vi "dareczkowe skalowanie.vi"(5 "nN":bool, 6 "um":bool, 7 "scaling in":dbl=1.37 format="%#_13g", 8 "amount to fit":dbl=0.5 format="%#_13g", 9 "all rows":dbl[][](array[numeric])) -> (0 "Contact Point index":i32, 1 "X":dbl[](array[numeric]), 2 "Y":dbl[](array[numeric]), 3 "Array":cluster{dbl[], dbl[]}[](array[cluster]), 4 "standard deviation":dbl format="%0.2f")   [LabVIEW 2015]
uses:
  <vilib>/Analysis/NI_AALBase.lvlib
  <vilib>/Analysis/NI_AALPro.lvlib
panel:
  out "Waveform Graph":dbl[](graph)
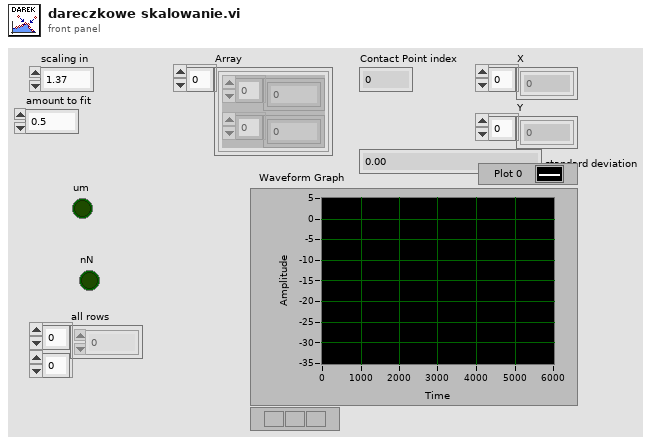
[diagram p1: front panel]
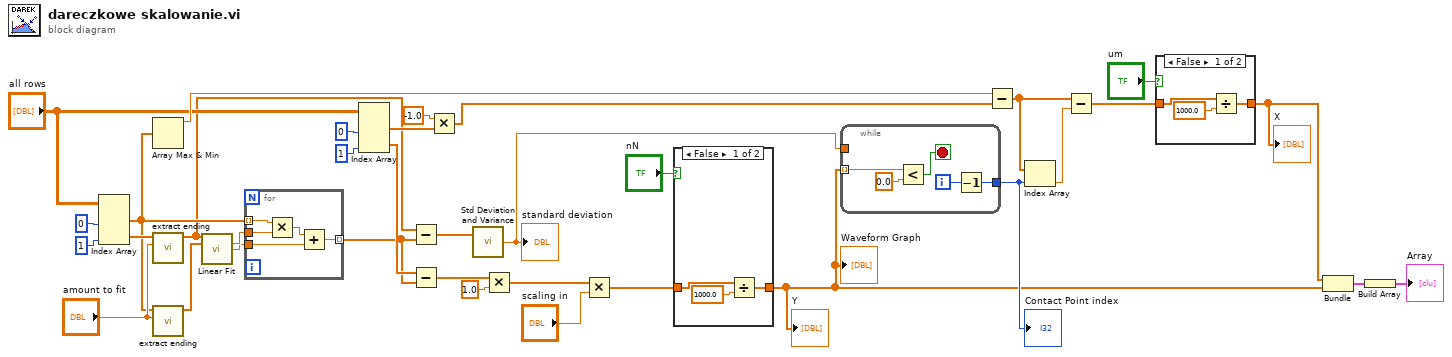
[diagram p0: block diagram]
diagram:
  n1 = Index Array(array="all rows", index (col) #1=0 ("disabled index (col)"), index (col) #2=1 ("index (col)")) -> (element #1=w15:dbl[], element #2=w20:dbl[])  [unwired: 2 in]
  n2 = Array Max & Min(array=w15) -> (max value=w33:dbl)  [unwired: 3 out]
  n3 = call "extract ending.vi"("length"="amount to fit", "all rows"=w20) -> ("Array"=w14:dbl[])  [unwired: 9 in]
  n4 = call "extract ending.vi"("length"="amount to fit", "all rows"=w15) -> ("Array"=w17:dbl[])  [unwired: 9 in]
  n5 = call <vilib>:"Linear Fit.vi"("Y"=w14, "X"=w17) -> ("slope"=w22:dbl, "intercept"=w21:dbl)  [unwired: 9 in, 3 out]
  n6 = for {
    tunnel: w15 -> [w36] mode=indexing
    tunnel: w22 -> [w38]
    tunnel: w21 -> [w39]
    tunnel: [w37] -> w12 mode=indexing
    n7 = Multiply(x=w36, y=w38) -> (x*y=w40:dbl)
    n8 = Add(x=w40, y=w39) -> (x+y=w37:dbl)
  }
  n9 = Index Array(array="all rows", index (col) #1=0 ("disabled index (col)"), index (col) #2=1 ("index (col)")) -> (element #1=w30:dbl[], element #2=w26:dbl[])  [unwired: 2 in]
  n10 = Subtract(x=w14, y=w12) -> (x-y=w13:dbl[])
  n11 = Subtract(x=w26, y=w12) -> (x-y=w11:dbl[])
  n12 = Multiply(x=-1.0, y=w30) -> (x*y=w35:dbl[])
  n13 = call <vilib>:"Std Deviation and Variance.vi"("X"=w13) -> ("standard deviation"=w10:dbl)  [unwired: 1 in, 2 out]
  "standard deviation" <- w10
  n14 = Multiply(x=w11, y=1.0) -> (x*y=w34:dbl[])
  n15 = Multiply(x=w34, y="scaling in") -> (x*y=w4:dbl[])
  n16 = case shown="False" "nN" {
    tunnel: [w42 w44] -> w3
    tunnel: w4 -> [w41 w44]
    frame False {
      n17 = Divide(x=w41, y=1000.0) -> (x/y=w42:dbl[])
    }
    frame True {
    }
  }
  "Y" <- w3
  "Waveform Graph" <- w3
  n18 = while {
    tunnel: w3 -> [w49] mode=indexing
    tunnel: w10 -> [_]
    tunnel: [w46] -> w9
    i -> [w45]
    stop <- w47 stop-if-true
    n19 = Less?(x=w49, y=0.0) -> (x < y?=w47:bool)
    n20 = Decrement(x=w45) -> (x-1=w46:i32)
  }
  "Contact Point index" <- w9
  n21 = Subtract(x=w33, y=w35) -> (x-y=w8:dbl[])
  n22 = Index Array(array=w8, index=w9) -> (element=w7:dbl)
  n23 = Subtract(x=w8, y=w7) -> (x-y=w6:dbl[])
  n24 = case shown="False" "um" {
    tunnel: [w51 w53] -> w5
    tunnel: w6 -> [w50 w53]
    frame False {
      n25 = Divide(x=w50, y=1000.0) -> (x/y=w51:dbl[])
    }
    frame True {
    }
  }
  "X" <- w5
  n26 = Bundle(w5, w3) -> (w29:cluster{dbl[], dbl[]})  [unwired: 1 in]
  n27 = Build Array(w29) -> (→"Array":cluster{dbl[], dbl[]}[])
